vi "MarbleDispenserMk9.vi"() -> ()   [LabVIEW 2016]
uses:
  <vilib>/NXT/Block Support/NXT_InputPort.ctl
  <vilib>/NXT/Block Support/NXT_OutputPort.ctl
  <vilib>/NXT/Dual Mode Library/Sensors/Touch_Released.vi
  <vilib>/NXT/NXTIO Xnodes/NXTIONodeSubVIs/NXTStopMotors.vi
  <vilib>/NXT/NXTIO Xnodes/NXTIONodeSubVIs/NXTMotorRunDistance.vi
  <vilib>/NXT/Dual Mode Library/Waits/Wait_Num.vi
  <vilib>/NXT/Dual Mode Library/Sensors/Touch_Pressed.vi
  <vilib>/NXT/Dual Mode Library/Sensors/EV3_Color_Color.vi
  <vilib>/NXT/Dual Mode Library/Sensors/EV3_Color_Reflect.vi
  <vilib>/NXT/Subs/LVHSConnector.ctl
  <vilib>/NXT/NXTIO Xnodes/AddressXNode/NXTIOAddress.xnode
  <vilib>/NXT/NXTIO Xnodes/NXTIOXNode/NXTIO.xnode
  <vilib>/NXT/LegoClasses/BrickReference/BrickReference.lvclass
panel:
  out "Size":string
  out "Speed":dbl
  out "Color":string
  out "Distance":dbl
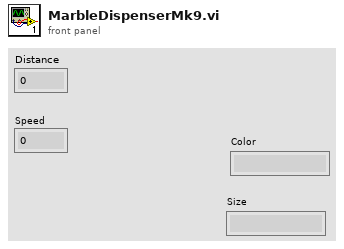
[diagram p1: front panel]
types:
  T1 = typedef "NXT_InputPort.ctl" = u32
  T2 = typedef "NXT_OutputPort.ctl" = u8
  T3 = typedef "LVHSConnector.ctl" = refnum<class "BrickReference.lvclass">
  T4 = typedef "ColorSensorColors.ctl" = enum16{"No Color", "Black", "Blue", "Green", "Yellow", "Red", "White", "Brown"}
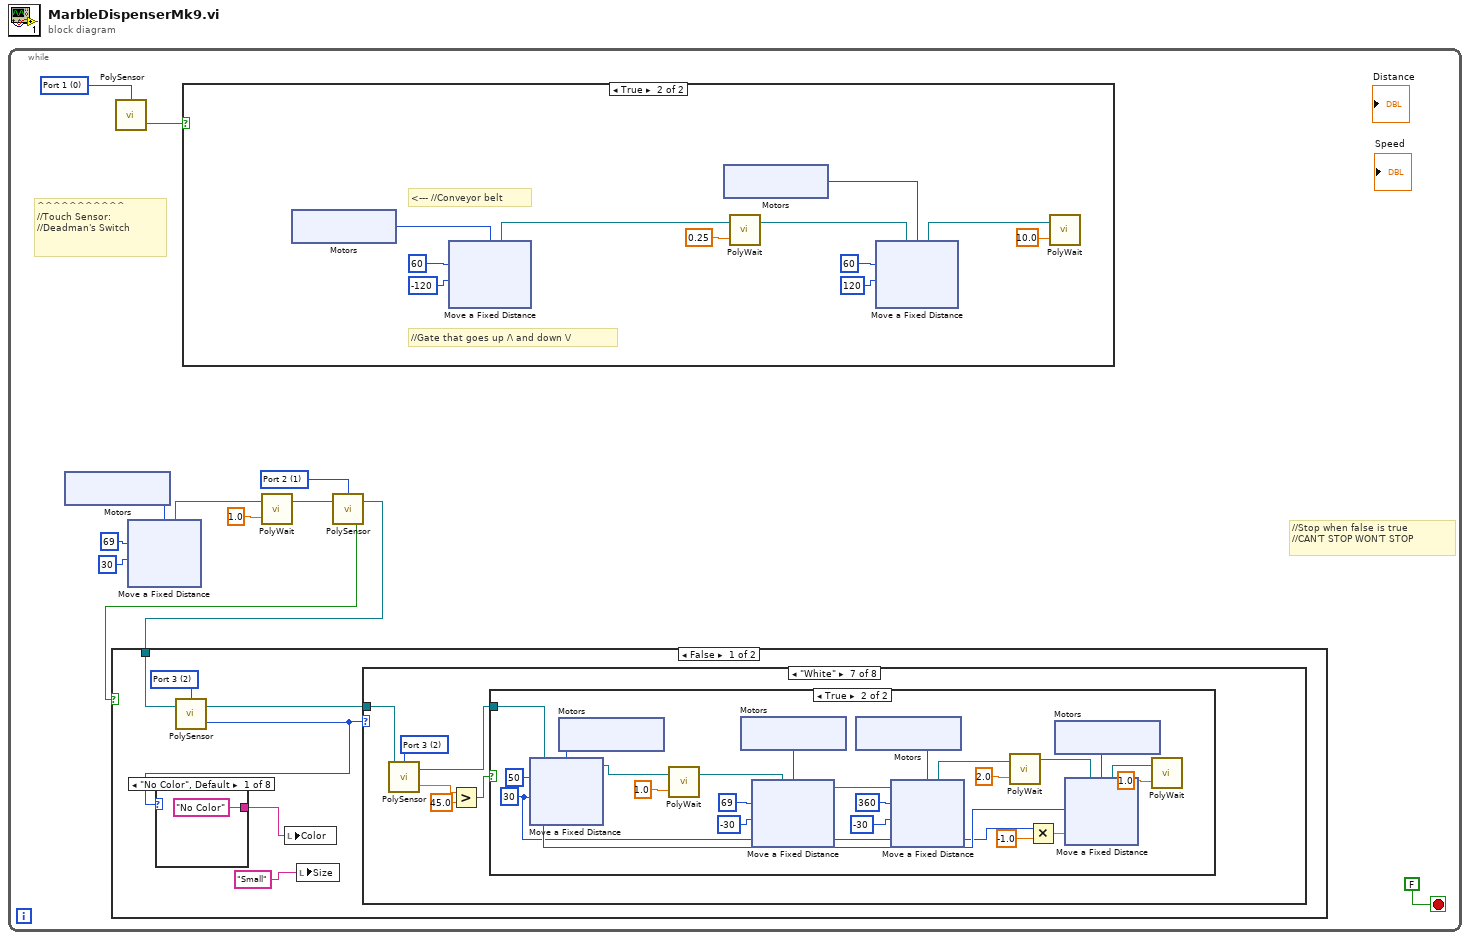
[diagram p0: block diagram]
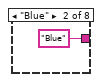
[diagram p2: hidden frame]
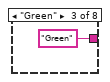
[diagram p3: hidden frame]
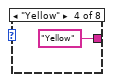
[diagram p4: hidden frame]
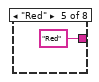
[diagram p5: hidden frame]
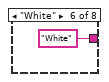
[diagram p6: hidden frame]
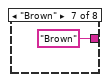
[diagram p7: hidden frame]
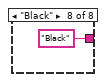
[diagram p8: hidden frame]
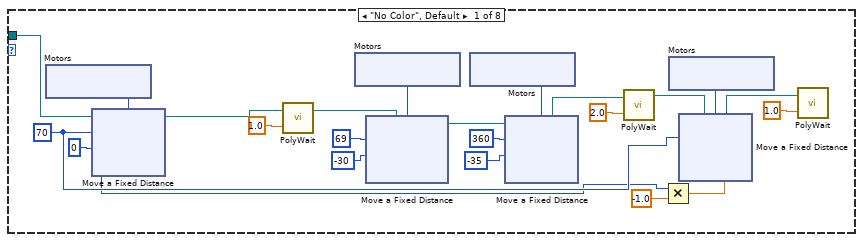
[diagram p9: hidden frame]
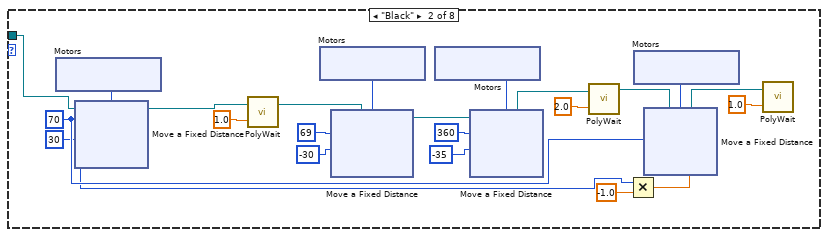
[diagram p10: hidden frame]
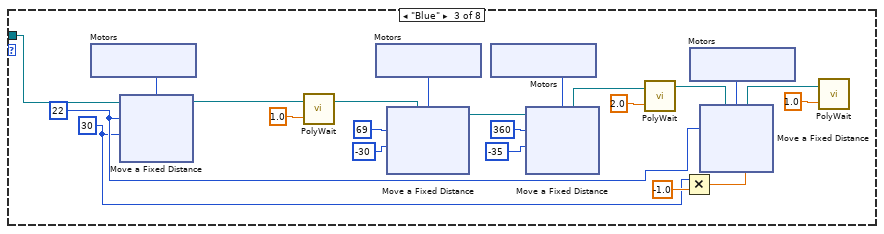
[diagram p11: hidden frame]
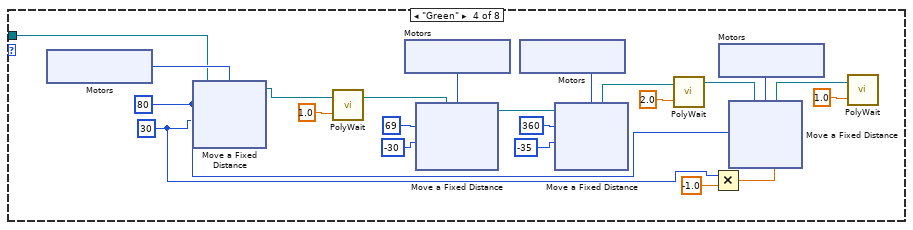
[diagram p12: hidden frame]
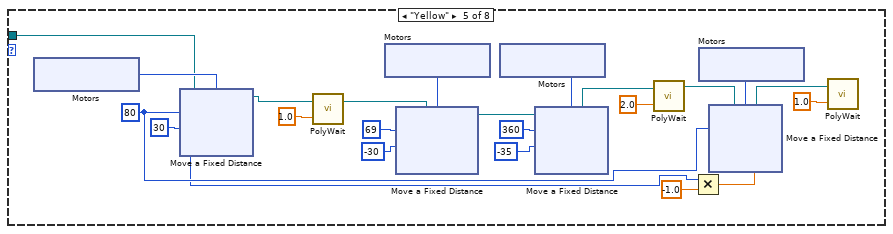
[diagram p13: hidden frame]
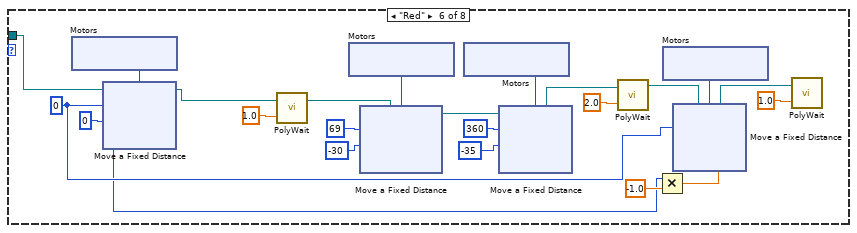
[diagram p14: hidden frame]
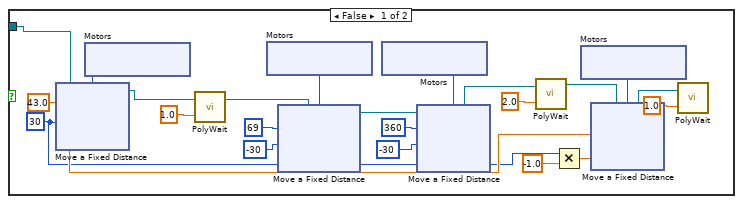
[diagram p15: hidden frame]
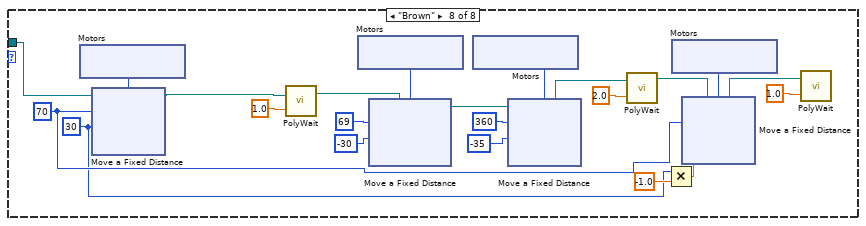
[diagram p16: hidden frame]
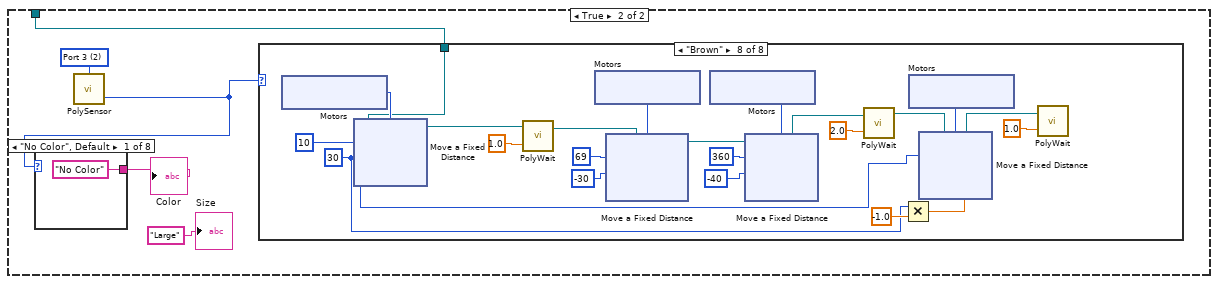
[diagram p17: hidden frame]
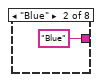
[diagram p18: hidden frame]
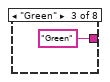
[diagram p19: hidden frame]
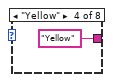
[diagram p20: hidden frame]
diagram:
  n1 = while {
    stop <- FALSE stop-if-true
    w3 = T1 1 items=["Port 1", "Port 2", "Port 3", "Port 4"] ("Port (Port 1)")
    w12 = T1 0 items=["Port 1", "Port 2", "Port 3", "Port 4"] ("Port (Port 1)")
    # "//Stop when false is true\n//CAN'T STOP WON'T STOP"
    # "^^^^^^^^^^^\n//Touch Sensor:\n//Deadman's Switch"
    n2 = xnode "Motors"() -> ("Motor"=w5:T2)
    n3 = call-poly <vilib>:"PolySensor.vi"("Port (Port 1)"=w12) -> ("Yes / No"=w10:bool)  [unwired: 2 in, 1 out]
    n4 = xnode "Move a Fixed Distance"("Speed 1"=30, "Distance 1"=69, "Motors"=w5) -> ("NXT/EV3"=w8:T3)  [unwired: 1 in]
    n5 = case shown="True" w10 {
      frame False {
        # "//This stops all the things"
        n6 = xnode "Motors"() -> ("Motor"=w1180:T2)
        n7 = xnode "Motors"() -> ("Motor"=w1179:T2)
        n8 = xnode "Stop Motors"("Motors"=w1180) -> ()  [unwired: 1 in, 1 out]
        n9 = xnode "Stop Motors"("Motors"=w1179) -> ()  [unwired: 1 in, 1 out]
      }
      frame True {
        # "//Gate that goes up /\\ and down \\/"
        # "<--- //Conveyor belt"
        n10 = xnode "Motors"() -> ("Motor"=w1199:T2)
        n11 = xnode "Move a Fixed Distance"("Speed 1"=-120, "Distance 1"=60, "Motors"=w1199) -> ("NXT/EV3"=w1202:T3)  [unwired: 1 in]
        n12 = xnode "Motors"() -> ("Motor"=w1193:T2)
        n13 = call-poly <vilib>:"PolyWait.vi"("Time (1 sec)"=0.25, "NXT/EV3"=w1202) -> ("NXT/EV3"=w1194:T3)  [unwired: 2 in]
        n14 = xnode "Move a Fixed Distance"("Speed 1"=120, "Distance 1"=60, "Motors"=w1193, "NXT/EV3"=w1194) -> ("NXT/EV3"=w1197:T3)
        n15 = call-poly <vilib>:"PolyWait.vi"("Time (1 sec)"=10.0, "NXT/EV3"=w1197) -> ()  [unwired: 2 in, 1 out]
      }
    }
    n16 = call-poly <vilib>:"PolyWait.vi"("Time (1 sec)"=1.0, "NXT/EV3"=w8) -> ("NXT/EV3"=w4:T3)  [unwired: 2 in]
    n17 = call-poly <vilib>:"PolySensor.vi"("NXT/EV3"=w4, "Port (Port 1)"=w3) -> ("Yes / No"=w2:bool, "NXT/EV3"=w1:T3)  [unwired: 1 in]
    n18 = case shown="False" w2 {
      tunnel: w1 -> [w15 w628]
      frame False {
        w18 = T1 2 items=["Port 1", "Port 2", "Port 3", "Port 4"] ("Port (Port 1)")
        n19 = call-poly <vilib>:"PolySensor.vi"("NXT/EV3"=w15, "Port (Port 1)"=w18) -> ("Detected Color"=w17:T4, "NXT/EV3"=w14:T3)  [unwired: 1 in]
        n20 = case shown="\"No Color\", Default" w17 {
          tunnel: ["No Color" "Blue" "Green" "Yellow" "Red" "White" "Brown" "Black"] -> w16
          frame "No Color", Default {
          }
          frame "Blue" {
          }
          frame "Green" {
          }
          frame "Yellow" {
          }
          frame "Red" {
          }
          frame "White" {
          }
          frame "Brown" {
          }
          frame "Black" {
          }
        }
        n21 = local write "Color"(w16) -> ()
        n22 = local write "Size"("Small") -> ()
        n23 = case shown="\"White\"" w17 {
          tunnel: w14 -> [w29 w96 w161 w228 w291 w377 w428 w561]
          frame "No Color", Default {
            w27 = i8 0 ("Speed 1")
            w28 = 70 ("Distance 1")
            n24 = xnode "Motors"() -> ("Motor"=w48:T2)
            n25 = xnode "Move a Fixed Distance"("Speed 1"=w27, "Distance 1"=w28, "Motors"=w48, "NXT/EV3"=w29) -> ("NXT/EV3"=w30:T3)
            n26 = call-poly <vilib>:"PolyWait.vi"("Time (1 sec)"=sgl 1.0, "NXT/EV3"=w30) -> ("NXT/EV3"=w43:T3)  [unwired: 2 in]
            n27 = xnode "Motors"() -> ("Motor"=w44:T2)
            n28 = xnode "Move a Fixed Distance"("Speed 1"=-30, "Distance 1"=69, "Motors"=w44, "NXT/EV3"=w43) -> ("NXT/EV3"=w33:T3)
            n29 = xnode "Motors"() -> ("Motor"=w40:T2)
            n30 = xnode "Move a Fixed Distance"("Speed 1"=i8 -35, "Distance 1"=360, "Motors"=w40, "NXT/EV3"=w33) -> ("NXT/EV3"=w41:T3)
            n31 = call-poly <vilib>:"PolyWait.vi"("Time (1 sec)"=2.0, "NXT/EV3"=w41) -> ("NXT/EV3"=w36:T3)  [unwired: 2 in]
            n32 = Multiply(x=w27, y=-1.0) -> (x*y=w31:dbl)
            n33 = xnode "Motors"() -> ("Motor"=w35:T2)
            n34 = xnode "Move a Fixed Distance"("Speed 1"=w31, "Distance 1"=w28, "Motors"=w35, "NXT/EV3"=w36) -> ("NXT/EV3"=w34:T3)
            n35 = call-poly <vilib>:"PolyWait.vi"("Time (1 sec)"=1.0, "NXT/EV3"=w34) -> ()  [unwired: 2 in, 1 out]
          }
          frame "Black" {
            w93 = i8 30 ("Speed 1")
            w94 = 70 ("Distance 1")
            n36 = xnode "Motors"() -> ("Motor"=w114:T2)
            n37 = xnode "Move a Fixed Distance"("Speed 1"=w93, "Distance 1"=w94, "Motors"=w114, "NXT/EV3"=w96) -> ("NXT/EV3"=w95:T3)
            n38 = call-poly <vilib>:"PolyWait.vi"("Time (1 sec)"=sgl 1.0, "NXT/EV3"=w95) -> ("NXT/EV3"=w109:T3)  [unwired: 2 in]
            n39 = xnode "Motors"() -> ("Motor"=w110:T2)
            n40 = xnode "Move a Fixed Distance"("Speed 1"=-30, "Distance 1"=69, "Motors"=w110, "NXT/EV3"=w109) -> ("NXT/EV3"=w99:T3)
            n41 = xnode "Motors"() -> ("Motor"=w106:T2)
            n42 = xnode "Move a Fixed Distance"("Speed 1"=i8 -35, "Distance 1"=360, "Motors"=w106, "NXT/EV3"=w99) -> ("NXT/EV3"=w107:T3)
            n43 = call-poly <vilib>:"PolyWait.vi"("Time (1 sec)"=2.0, "NXT/EV3"=w107) -> ("NXT/EV3"=w102:T3)  [unwired: 2 in]
            n44 = Multiply(x=w93, y=-1.0) -> (x*y=w97:dbl)
            n45 = xnode "Motors"() -> ("Motor"=w101:T2)
            n46 = xnode "Move a Fixed Distance"("Speed 1"=w97, "Distance 1"=w94, "Motors"=w101, "NXT/EV3"=w102) -> ("NXT/EV3"=w100:T3)
            n47 = call-poly <vilib>:"PolyWait.vi"("Time (1 sec)"=1.0, "NXT/EV3"=w100) -> ()  [unwired: 2 in, 1 out]
          }
          frame "Blue" {
            w159 = i8 30 ("Speed 1")
            w160 = 22 ("Distance 1")
            n48 = xnode "Motors"() -> ("Motor"=w180:T2)
            n49 = xnode "Move a Fixed Distance"("Speed 1"=w159, "Distance 1"=w160, "Motors"=w180, "NXT/EV3"=w161) -> ("NXT/EV3"=w162:T3)
            n50 = call-poly <vilib>:"PolyWait.vi"("Time (1 sec)"=sgl 1.0, "NXT/EV3"=w162) -> ("NXT/EV3"=w175:T3)  [unwired: 2 in]
            n51 = xnode "Motors"() -> ("Motor"=w176:T2)
            n52 = xnode "Move a Fixed Distance"("Speed 1"=-30, "Distance 1"=69, "Motors"=w176, "NXT/EV3"=w175) -> ("NXT/EV3"=w165:T3)
            n53 = xnode "Motors"() -> ("Motor"=w172:T2)
            n54 = xnode "Move a Fixed Distance"("Speed 1"=i8 -35, "Distance 1"=360, "Motors"=w172, "NXT/EV3"=w165) -> ("NXT/EV3"=w173:T3)
            n55 = call-poly <vilib>:"PolyWait.vi"("Time (1 sec)"=2.0, "NXT/EV3"=w173) -> ("NXT/EV3"=w168:T3)  [unwired: 2 in]
            n56 = Multiply(x=w159, y=-1.0) -> (x*y=w163:dbl)
            n57 = xnode "Motors"() -> ("Motor"=w167:T2)
            n58 = xnode "Move a Fixed Distance"("Speed 1"=w163, "Distance 1"=w160, "Motors"=w167, "NXT/EV3"=w168) -> ("NXT/EV3"=w166:T3)
            n59 = call-poly <vilib>:"PolyWait.vi"("Time (1 sec)"=1.0, "NXT/EV3"=w166) -> ()  [unwired: 2 in, 1 out]
          }
          frame "Green" {
            w225 = i8 30 ("Speed 1")
            w226 = 80 ("Distance 1")
            n60 = xnode "Motors"() -> ("Motor"=w246:T2)
            n61 = xnode "Move a Fixed Distance"("Speed 1"=w225, "Distance 1"=w226, "Motors"=w246, "NXT/EV3"=w228) -> ("NXT/EV3"=w227:T3)
            n62 = call-poly <vilib>:"PolyWait.vi"("Time (1 sec)"=sgl 1.0, "NXT/EV3"=w227) -> ("NXT/EV3"=w241:T3)  [unwired: 2 in]
            n63 = xnode "Motors"() -> ("Motor"=w242:T2)
            n64 = xnode "Move a Fixed Distance"("Speed 1"=-30, "Distance 1"=69, "Motors"=w242, "NXT/EV3"=w241) -> ("NXT/EV3"=w231:T3)
            n65 = xnode "Motors"() -> ("Motor"=w238:T2)
            n66 = xnode "Move a Fixed Distance"("Speed 1"=i8 -35, "Distance 1"=360, "Motors"=w238, "NXT/EV3"=w231) -> ("NXT/EV3"=w239:T3)
            n67 = call-poly <vilib>:"PolyWait.vi"("Time (1 sec)"=2.0, "NXT/EV3"=w239) -> ("NXT/EV3"=w234:T3)  [unwired: 2 in]
            n68 = Multiply(x=w225, y=-1.0) -> (x*y=w229:dbl)
            n69 = xnode "Motors"() -> ("Motor"=w233:T2)
            n70 = xnode "Move a Fixed Distance"("Speed 1"=w229, "Distance 1"=w226, "Motors"=w233, "NXT/EV3"=w234) -> ("NXT/EV3"=w232:T3)
            n71 = call-poly <vilib>:"PolyWait.vi"("Time (1 sec)"=1.0, "NXT/EV3"=w232) -> ()  [unwired: 2 in, 1 out]
          }
          frame "Yellow" {
            w292 = i8 30 ("Speed 1")
            w293 = 80 ("Distance 1")
            n72 = xnode "Motors"() -> ("Motor"=w312:T2)
            n73 = xnode "Move a Fixed Distance"("Speed 1"=w292, "Distance 1"=w293, "Motors"=w312, "NXT/EV3"=w291) -> ("NXT/EV3"=w294:T3)
            n74 = call-poly <vilib>:"PolyWait.vi"("Time (1 sec)"=sgl 1.0, "NXT/EV3"=w294) -> ("NXT/EV3"=w307:T3)  [unwired: 2 in]
            n75 = xnode "Motors"() -> ("Motor"=w308:T2)
            n76 = xnode "Move a Fixed Distance"("Speed 1"=-30, "Distance 1"=69, "Motors"=w308, "NXT/EV3"=w307) -> ("NXT/EV3"=w297:T3)
            n77 = xnode "Motors"() -> ("Motor"=w304:T2)
            n78 = xnode "Move a Fixed Distance"("Speed 1"=i8 -35, "Distance 1"=360, "Motors"=w304, "NXT/EV3"=w297) -> ("NXT/EV3"=w305:T3)
            n79 = call-poly <vilib>:"PolyWait.vi"("Time (1 sec)"=2.0, "NXT/EV3"=w305) -> ("NXT/EV3"=w300:T3)  [unwired: 2 in]
            n80 = Multiply(x=w292, y=-1.0) -> (x*y=w295:dbl)
            n81 = xnode "Motors"() -> ("Motor"=w299:T2)
            n82 = xnode "Move a Fixed Distance"("Speed 1"=w295, "Distance 1"=w293, "Motors"=w299, "NXT/EV3"=w300) -> ("NXT/EV3"=w298:T3)
            n83 = call-poly <vilib>:"PolyWait.vi"("Time (1 sec)"=1.0, "NXT/EV3"=w298) -> ()  [unwired: 2 in, 1 out]
          }
          frame "Red" {
            w357 = i8 0 ("Speed 1")
            w358 = 0 ("Distance 1")
            n84 = xnode "Motors"() -> ("Motor"=w378:T2)
            n85 = xnode "Move a Fixed Distance"("Speed 1"=w357, "Distance 1"=w358, "Motors"=w378, "NXT/EV3"=w377) -> ("NXT/EV3"=w359:T3)
            n86 = call-poly <vilib>:"PolyWait.vi"("Time (1 sec)"=sgl 1.0, "NXT/EV3"=w359) -> ("NXT/EV3"=w372:T3)  [unwired: 2 in]
            n87 = xnode "Motors"() -> ("Motor"=w373:T2)
            n88 = xnode "Move a Fixed Distance"("Speed 1"=-30, "Distance 1"=69, "Motors"=w373, "NXT/EV3"=w372) -> ("NXT/EV3"=w362:T3)
            n89 = xnode "Motors"() -> ("Motor"=w369:T2)
            n90 = xnode "Move a Fixed Distance"("Speed 1"=i8 -35, "Distance 1"=360, "Motors"=w369, "NXT/EV3"=w362) -> ("NXT/EV3"=w370:T3)
            n91 = call-poly <vilib>:"PolyWait.vi"("Time (1 sec)"=2.0, "NXT/EV3"=w370) -> ("NXT/EV3"=w365:T3)  [unwired: 2 in]
            n92 = Multiply(x=w357, y=-1.0) -> (x*y=w360:dbl)
            n93 = xnode "Motors"() -> ("Motor"=w364:T2)
            n94 = xnode "Move a Fixed Distance"("Speed 1"=w360, "Distance 1"=w358, "Motors"=w364, "NXT/EV3"=w365) -> ("NXT/EV3"=w363:T3)
            n95 = call-poly <vilib>:"PolyWait.vi"("Time (1 sec)"=1.0, "NXT/EV3"=w363) -> ()  [unwired: 2 in, 1 out]
          }
          frame "White" {
            w426 = T1 2 items=["Port 1", "Port 2", "Port 3", "Port 4"] ("Port (Port 1)")
            n96 = call-poly <vilib>:"PolySensor.vi"("NXT/EV3"=w428, "Port (Port 1)"=w426) -> ("Scaled Value"=w425:sgl, "NXT/EV3"=w427:T3)  [unwired: 1 in]
            n97 = Greater?(x=w425, y=sgl 45.0) -> (0:w423:bool)
            n98 = case shown="True" w423 {
              tunnel: w427 -> [w429 w515]
              frame False {
                w430 = i8 30 ("Speed 1")
                w431 = 43.0 ("Distance 1")
                n99 = xnode "Motors"() -> ("Motor"=w450:T2)
                n100 = xnode "Move a Fixed Distance"("Speed 1"=w430, "Distance 1"=w431, "Motors"=w450, "NXT/EV3"=w429) -> ("NXT/EV3"=w432:T3)
                n101 = call-poly <vilib>:"PolyWait.vi"("Time (1 sec)"=sgl 1.0, "NXT/EV3"=w432) -> ("NXT/EV3"=w445:T3)  [unwired: 2 in]
                n102 = xnode "Motors"() -> ("Motor"=w446:T2)
                n103 = xnode "Move a Fixed Distance"("Speed 1"=-30, "Distance 1"=69, "Motors"=w446, "NXT/EV3"=w445) -> ("NXT/EV3"=w435:T3)
                n104 = xnode "Motors"() -> ("Motor"=w442:T2)
                n105 = xnode "Move a Fixed Distance"("Speed 1"=i8 -30, "Distance 1"=360, "Motors"=w442, "NXT/EV3"=w435) -> ("NXT/EV3"=w443:T3)
                n106 = call-poly <vilib>:"PolyWait.vi"("Time (1 sec)"=2.0, "NXT/EV3"=w443) -> ("NXT/EV3"=w438:T3)  [unwired: 2 in]
                n107 = Multiply(x=w430, y=-1.0) -> (x*y=w433:dbl)
                n108 = xnode "Motors"() -> ("Motor"=w437:T2)
                n109 = xnode "Move a Fixed Distance"("Speed 1"=w433, "Distance 1"=w431, "Motors"=w437, "NXT/EV3"=w438) -> ("NXT/EV3"=w436:T3)
                n110 = call-poly <vilib>:"PolyWait.vi"("Time (1 sec)"=1.0, "NXT/EV3"=w436) -> ()  [unwired: 2 in, 1 out]
              }
              frame True {
                w495 = i8 30 ("Speed 1")
                w496 = 50 ("Distance 1")
                n111 = xnode "Motors"() -> ("Motor"=w516:T2)
                n112 = xnode "Move a Fixed Distance"("Speed 1"=w495, "Distance 1"=w496, "Motors"=w516, "NXT/EV3"=w515) -> ("NXT/EV3"=w497:T3)
                n113 = call-poly <vilib>:"PolyWait.vi"("Time (1 sec)"=sgl 1.0, "NXT/EV3"=w497) -> ("NXT/EV3"=w510:T3)  [unwired: 2 in]
                n114 = xnode "Motors"() -> ("Motor"=w511:T2)
                n115 = xnode "Move a Fixed Distance"("Speed 1"=-30, "Distance 1"=69, "Motors"=w511, "NXT/EV3"=w510) -> ("NXT/EV3"=w500:T3)
                n116 = xnode "Motors"() -> ("Motor"=w507:T2)
                n117 = xnode "Move a Fixed Distance"("Speed 1"=i8 -30, "Distance 1"=360, "Motors"=w507, "NXT/EV3"=w500) -> ("NXT/EV3"=w508:T3)
                n118 = call-poly <vilib>:"PolyWait.vi"("Time (1 sec)"=2.0, "NXT/EV3"=w508) -> ("NXT/EV3"=w503:T3)  [unwired: 2 in]
                n119 = Multiply(x=w495, y=-1.0) -> (x*y=w498:dbl)
                n120 = xnode "Motors"() -> ("Motor"=w502:T2)
                n121 = xnode "Move a Fixed Distance"("Speed 1"=w498, "Distance 1"=w496, "Motors"=w502, "NXT/EV3"=w503) -> ("NXT/EV3"=w501:T3)
                n122 = call-poly <vilib>:"PolyWait.vi"("Time (1 sec)"=1.0, "NXT/EV3"=w501) -> ()  [unwired: 2 in, 1 out]
              }
            }
          }
          frame "Brown" {
            w562 = i8 30 ("Speed 1")
            w563 = 70 ("Distance 1")
            n123 = xnode "Motors"() -> ("Motor"=w582:T2)
            n124 = xnode "Move a Fixed Distance"("Speed 1"=w562, "Distance 1"=w563, "Motors"=w582, "NXT/EV3"=w561) -> ("NXT/EV3"=w564:T3)
            n125 = call-poly <vilib>:"PolyWait.vi"("Time (1 sec)"=sgl 1.0, "NXT/EV3"=w564) -> ("NXT/EV3"=w577:T3)  [unwired: 2 in]
            n126 = xnode "Motors"() -> ("Motor"=w578:T2)
            n127 = xnode "Move a Fixed Distance"("Speed 1"=-30, "Distance 1"=69, "Motors"=w578, "NXT/EV3"=w577) -> ("NXT/EV3"=w567:T3)
            n128 = xnode "Motors"() -> ("Motor"=w574:T2)
            n129 = xnode "Move a Fixed Distance"("Speed 1"=i8 -35, "Distance 1"=360, "Motors"=w574, "NXT/EV3"=w567) -> ("NXT/EV3"=w575:T3)
            n130 = call-poly <vilib>:"PolyWait.vi"("Time (1 sec)"=2.0, "NXT/EV3"=w575) -> ("NXT/EV3"=w570:T3)  [unwired: 2 in]
            n131 = Multiply(x=w562, y=-1.0) -> (x*y=w565:dbl)
            n132 = xnode "Motors"() -> ("Motor"=w569:T2)
            n133 = xnode "Move a Fixed Distance"("Speed 1"=w565, "Distance 1"=w563, "Motors"=w569, "NXT/EV3"=w570) -> ("NXT/EV3"=w568:T3)
            n134 = call-poly <vilib>:"PolyWait.vi"("Time (1 sec)"=1.0, "NXT/EV3"=w568) -> ()  [unwired: 2 in, 1 out]
          }
        }
      }
      frame True {
        w631 = T1 2 items=["Port 1", "Port 2", "Port 3", "Port 4"] ("Port (Port 1)")
        n135 = call-poly <vilib>:"PolySensor.vi"("Port (Port 1)"=w631) -> ("Detected Color"=w629:T4)  [unwired: 2 in, 1 out]
        n136 = case shown="\"No Color\", Default" w629 {
          tunnel: ["No Color" "Blue" "Green" "Yellow" "Red" "White" "Brown" "Black"] -> w630
          frame "No Color", Default {
          }
          frame "Blue" {
          }
          frame "Green" {
          }
          frame "Yellow" {
          }
          frame "Red" {
          }
          frame "White" {
          }
          frame "Brown" {
          }
          frame "Black" {
          }
        }
        "Color" <- w630
        n137 = case shown="\"Brown\"" w629 {
          tunnel: w628 -> [w642 w708 w792 w858 w906 w990 w1038 w1104]
          frame "No Color", Default {
            w640 = i8 0 ("Speed 1")
            w641 = 0 ("Distance 1")
            n138 = xnode "Motors"() -> ("Motor"=w661:T2)
            n139 = xnode "Move a Fixed Distance"("Speed 1"=w640, "Distance 1"=w641, "Motors"=w661, "NXT/EV3"=w642) -> ("NXT/EV3"=w643:T3)
            n140 = call-poly <vilib>:"PolyWait.vi"("Time (1 sec)"=sgl 1.0, "NXT/EV3"=w643) -> ("NXT/EV3"=w656:T3)  [unwired: 2 in]
            n141 = xnode "Motors"() -> ("Motor"=w657:T2)
            n142 = xnode "Move a Fixed Distance"("Speed 1"=-30, "Distance 1"=69, "Motors"=w657, "NXT/EV3"=w656) -> ("NXT/EV3"=w646:T3)
            n143 = xnode "Motors"() -> ("Motor"=w653:T2)
            n144 = xnode "Move a Fixed Distance"("Speed 1"=i8 -40, "Distance 1"=360, "Motors"=w653, "NXT/EV3"=w646) -> ("NXT/EV3"=w654:T3)
            n145 = call-poly <vilib>:"PolyWait.vi"("Time (1 sec)"=2.0, "NXT/EV3"=w654) -> ("NXT/EV3"=w649:T3)  [unwired: 2 in]
            n146 = Multiply(x=w640, y=-1.0) -> (x*y=w644:dbl)
            n147 = xnode "Motors"() -> ("Motor"=w648:T2)
            n148 = xnode "Move a Fixed Distance"("Speed 1"=w644, "Distance 1"=w641, "Motors"=w648, "NXT/EV3"=w649) -> ("NXT/EV3"=w647:T3)
            n149 = call-poly <vilib>:"PolyWait.vi"("Time (1 sec)"=1.0, "NXT/EV3"=w647) -> ()  [unwired: 2 in, 1 out]
          }
          frame "Black" {
            w706 = i8 30 ("Speed 1")
            w707 = 10 ("Distance 1")
            n150 = xnode "Motors"() -> ("Motor"=w727:T2)
            n151 = xnode "Move a Fixed Distance"("Speed 1"=w706, "Distance 1"=w707, "Motors"=w727, "NXT/EV3"=w708) -> ("NXT/EV3"=w709:T3)
            n152 = call-poly <vilib>:"PolyWait.vi"("Time (1 sec)"=sgl 1.0, "NXT/EV3"=w709) -> ("NXT/EV3"=w722:T3)  [unwired: 2 in]
            n153 = xnode "Motors"() -> ("Motor"=w723:T2)
            n154 = xnode "Move a Fixed Distance"("Speed 1"=-30, "Distance 1"=69, "Motors"=w723, "NXT/EV3"=w722) -> ("NXT/EV3"=w712:T3)
            n155 = xnode "Motors"() -> ("Motor"=w719:T2)
            n156 = xnode "Move a Fixed Distance"("Speed 1"=i8 -40, "Distance 1"=360, "Motors"=w719, "NXT/EV3"=w712) -> ("NXT/EV3"=w720:T3)
            n157 = call-poly <vilib>:"PolyWait.vi"("Time (1 sec)"=2.0, "NXT/EV3"=w720) -> ("NXT/EV3"=w715:T3)  [unwired: 2 in]
            n158 = Multiply(x=w706, y=-1.0) -> (x*y=w710:dbl)
            n159 = xnode "Motors"() -> ("Motor"=w714:T2)
            n160 = xnode "Move a Fixed Distance"("Speed 1"=w710, "Distance 1"=w707, "Motors"=w714, "NXT/EV3"=w715) -> ("NXT/EV3"=w713:T3)
            n161 = call-poly <vilib>:"PolyWait.vi"("Time (1 sec)"=1.0, "NXT/EV3"=w713) -> ()  [unwired: 2 in, 1 out]
          }
          frame "Blue" {
            w772 = i8 30 ("Speed 1")
            w773 = 32 ("Distance 1")
            n162 = xnode "Motors"() -> ("Motor"=w793:T2)
            n163 = xnode "Move a Fixed Distance"("Speed 1"=w772, "Distance 1"=w773, "Motors"=w793, "NXT/EV3"=w792) -> ("NXT/EV3"=w774:T3)
            n164 = call-poly <vilib>:"PolyWait.vi"("Time (1 sec)"=sgl 1.0, "NXT/EV3"=w774) -> ("NXT/EV3"=w787:T3)  [unwired: 2 in]
            n165 = xnode "Motors"() -> ("Motor"=w788:T2)
            n166 = xnode "Move a Fixed Distance"("Speed 1"=-30, "Distance 1"=69, "Motors"=w788, "NXT/EV3"=w787) -> ("NXT/EV3"=w777:T3)
            n167 = xnode "Motors"() -> ("Motor"=w784:T2)
            n168 = xnode "Move a Fixed Distance"("Speed 1"=i8 -40, "Distance 1"=360, "Motors"=w784, "NXT/EV3"=w777) -> ("NXT/EV3"=w785:T3)
            n169 = call-poly <vilib>:"PolyWait.vi"("Time (1 sec)"=2.0, "NXT/EV3"=w785) -> ("NXT/EV3"=w780:T3)  [unwired: 2 in]
            n170 = Multiply(x=w772, y=-1.0) -> (x*y=w775:dbl)
            n171 = xnode "Motors"() -> ("Motor"=w779:T2)
            n172 = xnode "Move a Fixed Distance"("Speed 1"=w775, "Distance 1"=w773, "Motors"=w779, "NXT/EV3"=w780) -> ("NXT/EV3"=w778:T3)
            n173 = call-poly <vilib>:"PolyWait.vi"("Time (1 sec)"=1.0, "NXT/EV3"=w778) -> ()  [unwired: 2 in, 1 out]
          }
          frame "Green" {
            w838 = i8 30 ("Speed 1")
            w839 = 80 ("Distance 1")
            n174 = xnode "Motors"() -> ("Motor"=w859:T2)
            n175 = xnode "Move a Fixed Distance"("Speed 1"=w838, "Distance 1"=w839, "Motors"=w859, "NXT/EV3"=w858) -> ("NXT/EV3"=w840:T3)
            n176 = call-poly <vilib>:"PolyWait.vi"("Time (1 sec)"=sgl 1.0, "NXT/EV3"=w840) -> ("NXT/EV3"=w853:T3)  [unwired: 2 in]
            n177 = xnode "Motors"() -> ("Motor"=w854:T2)
            n178 = xnode "Move a Fixed Distance"("Speed 1"=-30, "Distance 1"=69, "Motors"=w854, "NXT/EV3"=w853) -> ("NXT/EV3"=w843:T3)
            n179 = xnode "Motors"() -> ("Motor"=w850:T2)
            n180 = xnode "Move a Fixed Distance"("Speed 1"=i8 -40, "Distance 1"=360, "Motors"=w850, "NXT/EV3"=w843) -> ("NXT/EV3"=w851:T3)
            n181 = call-poly <vilib>:"PolyWait.vi"("Time (1 sec)"=2.0, "NXT/EV3"=w851) -> ("NXT/EV3"=w846:T3)  [unwired: 2 in]
            n182 = Multiply(x=w838, y=-1.0) -> (x*y=w841:dbl)
            n183 = xnode "Motors"() -> ("Motor"=w845:T2)
            n184 = xnode "Move a Fixed Distance"("Speed 1"=w841, "Distance 1"=w839, "Motors"=w845, "NXT/EV3"=w846) -> ("NXT/EV3"=w844:T3)
            n185 = call-poly <vilib>:"PolyWait.vi"("Time (1 sec)"=1.0, "NXT/EV3"=w844) -> ()  [unwired: 2 in, 1 out]
          }
          frame "Yellow" {
            w904 = i8 30 ("Speed 1")
            w905 = 80 ("Distance 1")
            n186 = xnode "Motors"() -> ("Motor"=w925:T2)
            n187 = xnode "Move a Fixed Distance"("Speed 1"=w904, "Distance 1"=w905, "Motors"=w925, "NXT/EV3"=w906) -> ("NXT/EV3"=w907:T3)
            n188 = call-poly <vilib>:"PolyWait.vi"("Time (1 sec)"=sgl 1.0, "NXT/EV3"=w907) -> ("NXT/EV3"=w920:T3)  [unwired: 2 in]
            n189 = xnode "Motors"() -> ("Motor"=w921:T2)
            n190 = xnode "Move a Fixed Distance"("Speed 1"=-30, "Distance 1"=69, "Motors"=w921, "NXT/EV3"=w920) -> ("NXT/EV3"=w910:T3)
            n191 = xnode "Motors"() -> ("Motor"=w917:T2)
            n192 = xnode "Move a Fixed Distance"("Speed 1"=i8 -40, "Distance 1"=360, "Motors"=w917, "NXT/EV3"=w910) -> ("NXT/EV3"=w918:T3)
            n193 = call-poly <vilib>:"PolyWait.vi"("Time (1 sec)"=2.0, "NXT/EV3"=w918) -> ("NXT/EV3"=w913:T3)  [unwired: 2 in]
            n194 = Multiply(x=w904, y=-1.0) -> (x*y=w908:dbl)
            n195 = xnode "Motors"() -> ("Motor"=w912:T2)
            n196 = xnode "Move a Fixed Distance"("Speed 1"=w908, "Distance 1"=w905, "Motors"=w912, "NXT/EV3"=w913) -> ("NXT/EV3"=w911:T3)
            n197 = call-poly <vilib>:"PolyWait.vi"("Time (1 sec)"=1.0, "NXT/EV3"=w911) -> ()  [unwired: 2 in, 1 out]
          }
          frame "Red" {
            w970 = i8 30 ("Speed 1")
            w971 = 10 ("Distance 1")
            n198 = xnode "Motors"() -> ("Motor"=w991:T2)
            n199 = xnode "Move a Fixed Distance"("Speed 1"=w970, "Distance 1"=w971, "Motors"=w991, "NXT/EV3"=w990) -> ("NXT/EV3"=w972:T3)
            n200 = call-poly <vilib>:"PolyWait.vi"("Time (1 sec)"=sgl 1.0, "NXT/EV3"=w972) -> ("NXT/EV3"=w985:T3)  [unwired: 2 in]
            n201 = xnode "Motors"() -> ("Motor"=w986:T2)
            n202 = xnode "Move a Fixed Distance"("Speed 1"=-30, "Distance 1"=69, "Motors"=w986, "NXT/EV3"=w985) -> ("NXT/EV3"=w975:T3)
            n203 = xnode "Motors"() -> ("Motor"=w982:T2)
            n204 = xnode "Move a Fixed Distance"("Speed 1"=i8 -40, "Distance 1"=360, "Motors"=w982, "NXT/EV3"=w975) -> ("NXT/EV3"=w983:T3)
            n205 = call-poly <vilib>:"PolyWait.vi"("Time (1 sec)"=2.0, "NXT/EV3"=w983) -> ("NXT/EV3"=w978:T3)  [unwired: 2 in]
            n206 = Multiply(x=w970, y=-1.0) -> (x*y=w973:dbl)
            n207 = xnode "Motors"() -> ("Motor"=w977:T2)
            n208 = xnode "Move a Fixed Distance"("Speed 1"=w973, "Distance 1"=w971, "Motors"=w977, "NXT/EV3"=w978) -> ("NXT/EV3"=w976:T3)
            n209 = call-poly <vilib>:"PolyWait.vi"("Time (1 sec)"=1.0, "NXT/EV3"=w976) -> ()  [unwired: 2 in, 1 out]
          }
          frame "White" {
            w1036 = i8 30 ("Speed 1")
            w1037 = 81 ("Distance 1")
            n210 = xnode "Motors"() -> ("Motor"=w1057:T2)
            n211 = xnode "Move a Fixed Distance"("Speed 1"=w1036, "Distance 1"=w1037, "Motors"=w1057, "NXT/EV3"=w1038) -> ("NXT/EV3"=w1039:T3)
            n212 = call-poly <vilib>:"PolyWait.vi"("Time (1 sec)"=sgl 1.0, "NXT/EV3"=w1039) -> ("NXT/EV3"=w1052:T3)  [unwired: 2 in]
            n213 = xnode "Motors"() -> ("Motor"=w1053:T2)
            n214 = xnode "Move a Fixed Distance"("Speed 1"=-30, "Distance 1"=69, "Motors"=w1053, "NXT/EV3"=w1052) -> ("NXT/EV3"=w1042:T3)
            n215 = xnode "Motors"() -> ("Motor"=w1049:T2)
            n216 = xnode "Move a Fixed Distance"("Speed 1"=i8 -40, "Distance 1"=360, "Motors"=w1049, "NXT/EV3"=w1042) -> ("NXT/EV3"=w1050:T3)
            n217 = call-poly <vilib>:"PolyWait.vi"("Time (1 sec)"=2.0, "NXT/EV3"=w1050) -> ("NXT/EV3"=w1045:T3)  [unwired: 2 in]
            n218 = Multiply(x=w1036, y=-1.0) -> (x*y=w1040:dbl)
            n219 = xnode "Motors"() -> ("Motor"=w1044:T2)
            n220 = xnode "Move a Fixed Distance"("Speed 1"=w1040, "Distance 1"=w1037, "Motors"=w1044, "NXT/EV3"=w1045) -> ("NXT/EV3"=w1043:T3)
            n221 = call-poly <vilib>:"PolyWait.vi"("Time (1 sec)"=1.0, "NXT/EV3"=w1043) -> ()  [unwired: 2 in, 1 out]
          }
          frame "Brown" {
            w1102 = i8 30 ("Speed 1")
            w1103 = 10 ("Distance 1")
            n222 = xnode "Motors"() -> ("Motor"=w1123:T2)
            n223 = xnode "Move a Fixed Distance"("Speed 1"=w1102, "Distance 1"=w1103, "Motors"=w1123, "NXT/EV3"=w1104) -> ("NXT/EV3"=w1105:T3)
            n224 = call-poly <vilib>:"PolyWait.vi"("Time (1 sec)"=sgl 1.0, "NXT/EV3"=w1105) -> ("NXT/EV3"=w1118:T3)  [unwired: 2 in]
            n225 = xnode "Motors"() -> ("Motor"=w1119:T2)
            n226 = xnode "Move a Fixed Distance"("Speed 1"=-30, "Distance 1"=69, "Motors"=w1119, "NXT/EV3"=w1118) -> ("NXT/EV3"=w1108:T3)
            n227 = xnode "Motors"() -> ("Motor"=w1115:T2)
            n228 = xnode "Move a Fixed Distance"("Speed 1"=i8 -40, "Distance 1"=360, "Motors"=w1115, "NXT/EV3"=w1108) -> ("NXT/EV3"=w1116:T3)
            n229 = call-poly <vilib>:"PolyWait.vi"("Time (1 sec)"=2.0, "NXT/EV3"=w1116) -> ("NXT/EV3"=w1111:T3)  [unwired: 2 in]
            n230 = Multiply(x=w1102, y=-1.0) -> (x*y=w1106:dbl)
            n231 = xnode "Motors"() -> ("Motor"=w1110:T2)
            n232 = xnode "Move a Fixed Distance"("Speed 1"=w1106, "Distance 1"=w1103, "Motors"=w1110, "NXT/EV3"=w1111) -> ("NXT/EV3"=w1109:T3)
            n233 = call-poly <vilib>:"PolyWait.vi"("Time (1 sec)"=1.0, "NXT/EV3"=w1109) -> ()  [unwired: 2 in, 1 out]
          }
        }
        "Size" <- "Large"
      }
    }
  }
